vi "guangzi_16_up2.vi"() -> ()   [LabVIEW 2016]
uses:
  <vilib>/Utility/file.llb/Write To Spreadsheet File (DBL).vi
panel:
  in  "选项卡控件":T1(tab)
  in  "对数":bool
  out "MCS8Dat Error":i32
  out "通道数":i32
  out "Data 9":dbl[](graph)
  out "MCS8Dat Error 2":i32
  out "通道数 2":i32
  in  "对数 2":bool
  out "Data10":dbl[](graph)
  out "MCS8Dat Error 3":i32
  out "通道数 3":i32
  in  "对数 3":bool
  out "Data10 2":dbl[](graph)
  out "MCS8Dat Error 4":i32
  out "通道数 4":i32
  in  "对数 4":bool
  out "Data10 3":dbl[](graph)
  out "MCS8Dat Error 5":i32
  out "通道数 5":i32
  in  "对数 5":bool
  out "Data10 4":dbl[](graph)
  out "MCS8Dat Error 6":i32
  out "通道数 6":i32
  in  "对数 6":bool
  out "Data10 5":dbl[](graph)
  out "MCS8Dat Error 7":i32
  out "通道数 7":i32
  in  "对数 7":bool
  out "Data10 6":dbl[](graph)
  out "MCS8Dat Error 8":i32
  out "通道数 8":i32
  in  "对数 8":bool
  out "Data10 7":dbl[](graph)
  out "MCS8Dat Error 9":i32
  out "通道数 9":i32
  in  "对数 9":bool
  out "Data108":dbl[](graph)
  in  "对数 10":bool
  out "通道数 10":i32
  out "MCS8Dat Error 10":i32
  out "Data10 9":dbl[](graph)
  in  "对数 11":bool
  out "通道数 11":i32
  out "MCS8Dat Error 11":i32
  out "Data10 10":dbl[](graph)
  in  "对数 12":bool
  out "通道数 12":i32
  out "MCS8Dat Error 12":i32
  out "Data10 11":dbl[](graph)
  in  "对数 13":bool
  out "通道数 13":i32
  out "MCS8Dat Error 13":i32
  out "Data10 12":dbl[](graph)
  in  "对数 14":bool
  out "通道数 14":i32
  out "MCS8Dat Error 14":i32
  out "Data10 13":dbl[](graph)
  in  "对数 15":bool
  out "通道数 15":i32
  out "MCS8Dat Error 15":i32
  out "Data10 14":dbl[](graph)
  in  "对数 16":bool
  out "通道数 16":i32
  out "MCS8Dat Error 16":i32
  out "Data10 15":dbl[](graph)
  in  "切片值":i32
  out "切片图":u32[](graph)
  in  "采集开关":bool
  in  "子开关":bool
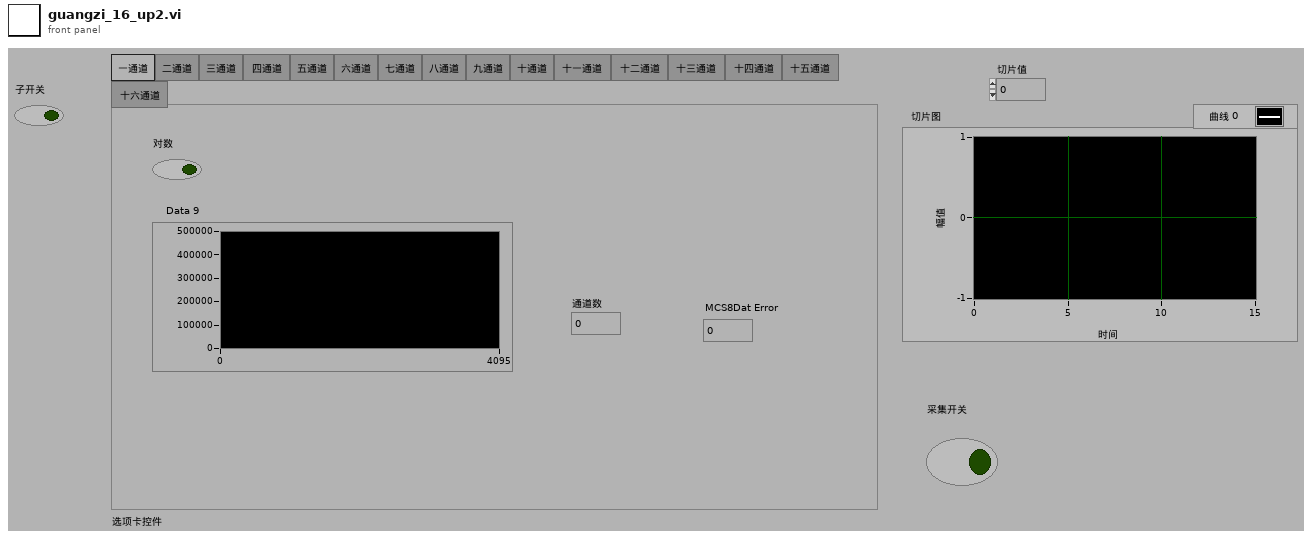
[diagram p1: front panel]
types:
  T1 = enum32{"一通道", "二通道", "三通道", "四通道 ", "五通道", "六通道", "七通道", "八通道", "九通道", "十通道", "十一通道 ", "十二通道 ", "十三通道 ", "十四通道 ", "十五通道 ", "十六通道 "}
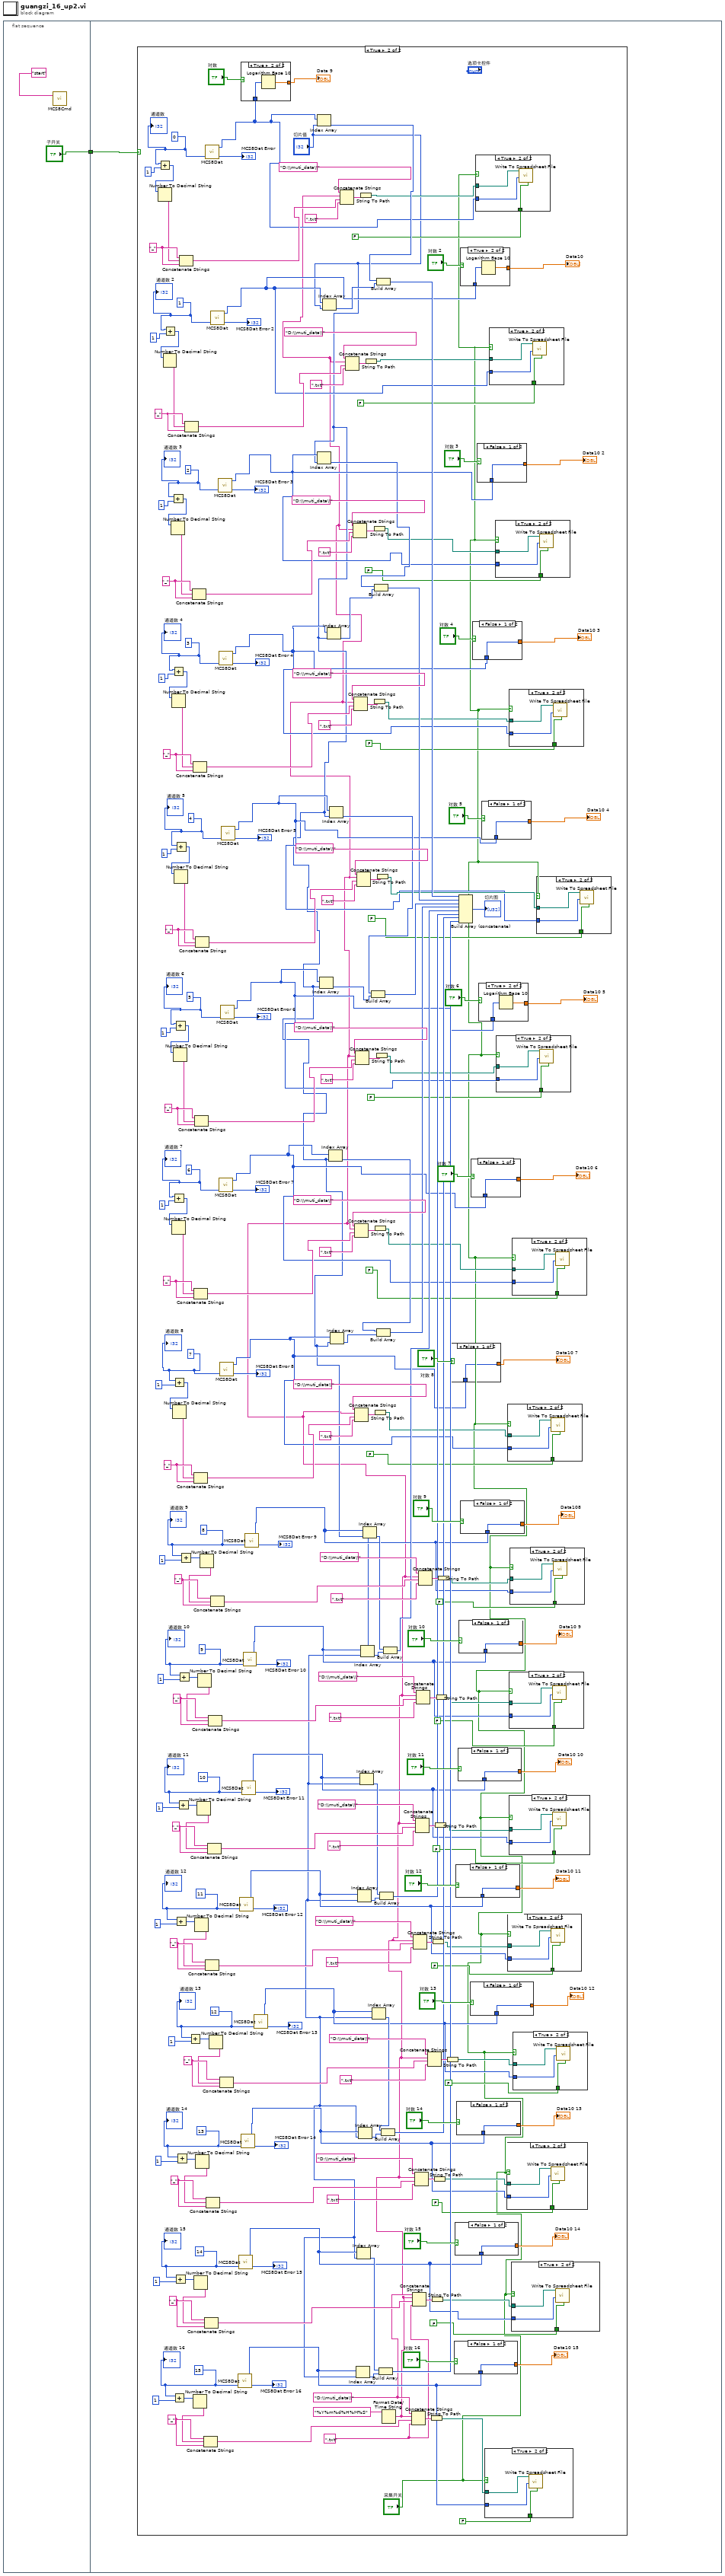
[diagram p0: block diagram]
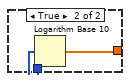
[diagram p19: hidden frame]
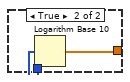
[diagram p20: hidden frame]
diagram:
  n1 = flat-sequence {
    tunnel: ["子开关"] -> w1
    tunnel: w1 -> [w4]
    frame #0 {
      n2 = call "MCS8Cmd.vi"("Command"="start") -> ()  [unwired: 2 in, 1 out]
    }
    frame #1 {
      n3 = case shown="True" w4 {
        frame False {
        }
        frame True {
          w6 = ".txt"
          w7 = "D:\\muti_data\\"
          w65 = "_"
          w69 = 15
          w75 = "_"
          w79 = 14
          w90 = "_"
          w94 = 13
          w102 = "_"
          w106 = 12
          w117 = "_"
          w121 = 11
          w129 = "_"
          w133 = 10
          w144 = "_"
          w148 = 9
          w156 = "_"
          w160 = 8
          w192 = 7
          w198 = "_"
          w202 = 6
          w208 = "_"
          w212 = 5
          w218 = "_"
          w222 = 4
          w228 = "_"
          w232 = 3
          w238 = "_"
          w242 = 2
          w248 = "_"
          w252 = 1
          w258 = "_"
          w262 = 0
          w268 = "_"
          n4 = Add(x=w262, y=1) -> (x+y=w264:i32)
          n5 = Number To Decimal String(number=w264) -> (decimal integer string=w267:string)  [unwired: 1 in]
          n6 = Add(x=w252, y=1) -> (x+y=w254:i32)
          n7 = Number To Decimal String(number=w254) -> (decimal integer string=w257:string)  [unwired: 1 in]
          n8 = Add(x=w242, y=1) -> (x+y=w244:i32)
          n9 = Number To Decimal String(number=w244) -> (decimal integer string=w247:string)  [unwired: 1 in]
          n10 = Add(x=w232, y=1) -> (x+y=w234:i32)
          n11 = Number To Decimal String(number=w234) -> (decimal integer string=w237:string)  [unwired: 1 in]
          n12 = Add(x=w202, y=1) -> (x+y=w204:i32)
          n13 = Number To Decimal String(number=w204) -> (decimal integer string=w207:string)  [unwired: 1 in]
          n14 = Add(x=w192, y=1) -> (x+y=w194:i32)
          n15 = Number To Decimal String(number=w194) -> (decimal integer string=w197:string)  [unwired: 1 in]
          n16 = Add(x=w69, y=1) -> (x+y=w70:i32)
          n17 = Add(x=w212, y=1) -> (x+y=w214:i32)
          n18 = Number To Decimal String(number=w214) -> (decimal integer string=w217:string)  [unwired: 1 in]
          n19 = Add(x=w79, y=1) -> (x+y=w80:i32)
          n20 = Add(x=w222, y=1) -> (x+y=w224:i32)
          n21 = Number To Decimal String(number=w224) -> (decimal integer string=w227:string)  [unwired: 1 in]
          n22 = Add(x=w121, y=1) -> (x+y=w122:i32)
          n23 = Add(x=w94, y=1) -> (x+y=w95:i32)
          n24 = Add(x=w133, y=1) -> (x+y=w134:i32)
          n25 = Add(x=w148, y=1) -> (x+y=w149:i32)
          n26 = Concatenate Strings(w268, w267, w268) -> (w266:string)
          n27 = Add(x=w160, y=1) -> (x+y=w161:i32)
          n28 = Concatenate Strings(w258, w257, w258) -> (w256:string)
          n29 = Add(x=w106, y=1) -> (x+y=w107:i32)
          n30 = Concatenate Strings(w248, w247, w248) -> (w246:string)
          n31 = Concatenate Strings(w238, w237, w238) -> (w236:string)
          n32 = Number To Decimal String(number=w70) -> (decimal integer string=w64:string)  [unwired: 1 in]
          n33 = Concatenate Strings(w208, w207, w208) -> (w206:string)
          n34 = Concatenate Strings(w198, w197, w198) -> (w196:string)
          n35 = Number To Decimal String(number=w80) -> (decimal integer string=w74:string)  [unwired: 1 in]
          n36 = Concatenate Strings(w218, w217, w218) -> (w216:string)
          n37 = Number To Decimal String(number=w122) -> (decimal integer string=w116:string)  [unwired: 1 in]
          n38 = Concatenate Strings(w228, w227, w228) -> (w226:string)
          n39 = Number To Decimal String(number=w95) -> (decimal integer string=w89:string)  [unwired: 1 in]
          n40 = Number To Decimal String(number=w134) -> (decimal integer string=w128:string)  [unwired: 1 in]
          n41 = Number To Decimal String(number=w149) -> (decimal integer string=w143:string)  [unwired: 1 in]
          n42 = Number To Decimal String(number=w161) -> (decimal integer string=w155:string)  [unwired: 1 in]
          n43 = Concatenate Strings(w65, w64, w65) -> (w62:string)
          n44 = Concatenate Strings(w75, w74, w75) -> (w73:string)
          n45 = call "MCS8Dat.vi"("Spectrum #"=w262) -> ("MCS8Dat Error"=→"MCS8Dat Error":i32, "Data"=w11:u32[])  [unwired: 2 in, 1 out]
          n46 = Concatenate Strings(w117, w116, w117) -> (w114:string)
          n47 = Concatenate Strings(w90, w89, w90) -> (w87:string)
          n48 = Concatenate Strings(w129, w128, w129) -> (w126:string)
          n49 = Concatenate Strings(w144, w143, w144) -> (w141:string)
          n50 = Number To Decimal String(number=w107) -> (decimal integer string=w101:string)  [unwired: 1 in]
          n51 = call "MCS8Dat.vi"("Spectrum #"=w252) -> ("MCS8Dat Error"=→"MCS8Dat Error 2":i32, "Data"=w14:u32[])  [unwired: 2 in, 1 out]
          n52 = Concatenate Strings(w156, w155, w156) -> (w153:string)
          n53 = call "MCS8Dat.vi"("Spectrum #"=w242) -> ("MCS8Dat Error"=→"MCS8Dat Error 3":i32, "Data"=w17:u32[])  [unwired: 2 in, 1 out]
          n54 = call "MCS8Dat.vi"("Spectrum #"=w232) -> ("MCS8Dat Error"=→"MCS8Dat Error 4":i32, "Data"=w20:u32[])  [unwired: 2 in, 1 out]
          n55 = call "MCS8Dat.vi"("Spectrum #"=w202) -> ("MCS8Dat Error"=→"MCS8Dat Error 7":i32, "Data"=w29:u32[])  [unwired: 2 in, 1 out]
          n56 = call "MCS8Dat.vi"("Spectrum #"=w192) -> ("MCS8Dat Error"=→"MCS8Dat Error 8":i32, "Data"=w32:u32[])  [unwired: 2 in, 1 out]
          n57 = Concatenate Strings(w102, w101, w102) -> (w99:string)
          n58 = call "MCS8Dat.vi"("Spectrum #"=w212) -> ("MCS8Dat Error"=→"MCS8Dat Error 6":i32, "Data"=w26:u32[])  [unwired: 2 in, 1 out]
          n59 = call "MCS8Dat.vi"("Spectrum #"=w222) -> ("MCS8Dat Error"=→"MCS8Dat Error 5":i32, "Data"=w23:u32[])  [unwired: 2 in, 1 out]
          n60 = call "MCS8Dat.vi"("Spectrum #"=w69) -> ("MCS8Dat Error"=→"MCS8Dat Error 16":i32, "Data"=w56:u32[])  [unwired: 2 in, 1 out]
          n61 = call "MCS8Dat.vi"("Spectrum #"=w79) -> ("MCS8Dat Error"=→"MCS8Dat Error 15":i32, "Data"=w53:u32[])  [unwired: 2 in, 1 out]
          n62 = call "MCS8Dat.vi"("Spectrum #"=w121) -> ("MCS8Dat Error"=→"MCS8Dat Error 12":i32, "Data"=w44:u32[])  [unwired: 2 in, 1 out]
          n63 = call "MCS8Dat.vi"("Spectrum #"=w94) -> ("MCS8Dat Error"=→"MCS8Dat Error 14":i32, "Data"=w50:u32[])  [unwired: 2 in, 1 out]
          n64 = case shown="True" "对数" {
            tunnel: w11 -> [w365 w366]
            tunnel: [w365 w367] -> w177
            frame False {
            }
            frame True {
              n65 = Logarithm Base 10(1:w366) -> (0:w367:dbl[])
            }
          }
          "Data 9" <- w177
          n66 = call "MCS8Dat.vi"("Spectrum #"=w133) -> ("MCS8Dat Error"=→"MCS8Dat Error 11":i32, "Data"=w41:u32[])  [unwired: 2 in, 1 out]
          n67 = call "MCS8Dat.vi"("Spectrum #"=w148) -> ("MCS8Dat Error"=→"MCS8Dat Error 10":i32, "Data"=w38:u32[])  [unwired: 2 in, 1 out]
          n68 = call "MCS8Dat.vi"("Spectrum #"=w160) -> ("MCS8Dat Error"=→"MCS8Dat Error 9":i32, "Data"=w35:u32[])  [unwired: 2 in, 1 out]
          n69 = call "MCS8Dat.vi"("Spectrum #"=w106) -> ("MCS8Dat Error"=→"MCS8Dat Error 13":i32, "Data"=w47:u32[])  [unwired: 2 in, 1 out]
          n70 = Index Array(array=w11, index="切片值") -> (element=w185:u32)
          n71 = Index Array(array=w17, index="切片值") -> (element=w187:u32)
          n72 = Index Array(array=w26, index="切片值") -> (element=w189:u32)
          n73 = Index Array(array=w14, index="切片值") -> (element=w184:u32)
          n74 = Index Array(array=w20, index="切片值") -> (element=w186:u32)
          n75 = Index Array(array=w29, index="切片值") -> (element=w190:u32)
          n76 = Index Array(array=w23, index="切片值") -> (element=w188:u32)
          n77 = Index Array(array=w32, index="切片值") -> (element=w191:u32)
          n78 = Index Array(array=w56, index="切片值") -> (element=w60:u32)
          n79 = Index Array(array=w53, index="切片值") -> (element=w59:u32)
          n80 = Index Array(array=w44, index="切片值") -> (element=w110:u32)
          n81 = Index Array(array=w50, index="切片值") -> (element=w83:u32)
          n82 = Index Array(array=w41, index="切片值") -> (element=w111:u32)
          n83 = Index Array(array=w38, index="切片值") -> (element=w137:u32)
          n84 = Index Array(array=w35, index="切片值") -> (element=w138:u32)
          n85 = Build Array(w188, w189) -> (w181:u32[])
          n86 = Index Array(array=w47, index="切片值") -> (element=w84:u32)
          n87 = Build Array(w187, w186) -> (w182:u32[])
          n88 = Build Array(w190, w191) -> (w180:u32[])
          n89 = Build Array(w185, w184) -> (w183:u32[])
          n90 = Build Array(w59, w60) -> (w58:u32[])
          n91 = Build Array(w111, w110) -> (w109:u32[])
          n92 = Build Array(w84, w83) -> (w82:u32[])
          n93 = Format Date/Time String(time format string (%c)="%Y%m%d%H%M%S") -> (date/time string=w5:string)  [unwired: 2 in]
          n94 = Concatenate Strings("D:\\muti_data\\", w5, w266, ".txt") -> (w270:string)
          n95 = Concatenate Strings("D:\\muti_data\\", w5, w256, ".txt") -> (w260:string)
          n96 = Concatenate Strings("D:\\muti_data\\", w5, w246, ".txt") -> (w250:string)
          n97 = Concatenate Strings("D:\\muti_data\\", w5, w236, ".txt") -> (w240:string)
          n98 = Concatenate Strings("D:\\muti_data\\", w5, w206, ".txt") -> (w210:string)
          n99 = Concatenate Strings("D:\\muti_data\\", w5, w196, ".txt") -> (w200:string)
          n100 = Concatenate Strings("D:\\muti_data\\", w5, w216, ".txt") -> (w220:string)
          n101 = Concatenate Strings("D:\\muti_data\\", w5, w226, ".txt") -> (w230:string)
          n102 = String To Path(string=w270) -> (path=w12:path)
          n103 = String To Path(string=w260) -> (path=w15:path)
          n104 = String To Path(string=w250) -> (path=w18:path)
          n105 = String To Path(string=w240) -> (path=w21:path)
          n106 = String To Path(string=w210) -> (path=w30:path)
          n107 = String To Path(string=w200) -> (path=w33:path)
          n108 = String To Path(string=w220) -> (path=w27:path)
          n109 = String To Path(string=w230) -> (path=w24:path)
          n110 = Build Array(w138, w137) -> (w136:u32[])
          n111 = Concatenate Strings(w7, w5, w62, w6) -> (w61:string)
          n112 = Concatenate Strings(w7, w5, w73, w6) -> (w72:string)
          n113 = Concatenate Strings("D:\\muti_data\\", w5, w114, ".txt") -> (w112:string)
          n114 = Concatenate Strings("D:\\muti_data\\", w5, w87, ".txt") -> (w85:string)
          n115 = Concatenate Strings("D:\\muti_data\\", w5, w126, ".txt") -> (w124:string)
          n116 = Concatenate Strings("D:\\muti_data\\", w5, w141, ".txt") -> (w139:string)
          n117 = Concatenate Strings("D:\\muti_data\\", w5, w153, ".txt") -> (w151:string)
          n118 = Concatenate Strings("D:\\muti_data\\", w5, w99, ".txt") -> (w97:string)
          n119 = String To Path(string=w61) -> (path=w57:path)
          n120 = String To Path(string=w72) -> (path=w54:path)
          n121 = String To Path(string=w112) -> (path=w45:path)
          n122 = String To Path(string=w85) -> (path=w49:path)
          n123 = String To Path(string=w124) -> (path=w42:path)
          n124 = String To Path(string=w139) -> (path=w39:path)
          n125 = String To Path(string=w151) -> (path=w36:path)
          n126 = String To Path(string=w97) -> (path=w48:path)
          n127 = case shown="False" "对数 8" {
            tunnel: w32 -> [w344 w346]
            tunnel: [w344 w345] -> w163
            frame False {
            }
            frame True {
              n128 = Logarithm Base 10(1:w346) -> (0:w345:dbl[])
            }
          }
          "Data10 7" <- w163
          n129 = case shown="False" "对数 16" {
            tunnel: w56 -> [w320 w322]
            tunnel: [w320 w321] -> w66
            frame False {
            }
            frame True {
              n130 = Logarithm Base 10(1:w322) -> (0:w321:dbl[])
            }
          }
          "Data10 15" <- w66
          n131 = case shown="False" "对数 15" {
            tunnel: w53 -> [w323 w325]
            tunnel: [w323 w324] -> w76
            frame False {
            }
            frame True {
              n132 = Logarithm Base 10(1:w325) -> (0:w324:dbl[])
            }
          }
          "Data10 14" <- w76
          n133 = case shown="False" "对数 12" {
            tunnel: w44 -> [w332 w334]
            tunnel: [w332 w333] -> w118
            frame False {
            }
            frame True {
              n134 = Logarithm Base 10(1:w334) -> (0:w333:dbl[])
            }
          }
          "Data10 11" <- w118
          n135 = case shown="False" "对数 14" {
            tunnel: w50 -> [w326 w328]
            tunnel: [w326 w327] -> w91
            frame False {
            }
            frame True {
              n136 = Logarithm Base 10(1:w328) -> (0:w327:dbl[])
            }
          }
          "Data10 13" <- w91
          n137 = case shown="False" "对数 11" {
            tunnel: w41 -> [w335 w337]
            tunnel: [w335 w336] -> w130
            frame False {
            }
            frame True {
              n138 = Logarithm Base 10(1:w337) -> (0:w336:dbl[])
            }
          }
          "Data10 10" <- w130
          n139 = Build Array (concatenate)(w183, w182, w181, w180, w136, w109, w82, w58) -> (→"切片图":u32[])
          n140 = case shown="False" "对数 10" {
            tunnel: w38 -> [w338 w340]
            tunnel: [w338 w339] -> w145
            frame False {
            }
            frame True {
              n141 = Logarithm Base 10(1:w340) -> (0:w339:dbl[])
            }
          }
          "Data10 9" <- w145
          n142 = case shown="True" "对数 2" {
            tunnel: w14 -> [w362 w364]
            tunnel: [w362 w363] -> w175
            frame False {
            }
            frame True {
              n143 = Logarithm Base 10(1:w364) -> (0:w363:dbl[])
            }
          }
          "Data10" <- w175
          n144 = case shown="False" "对数 9" {
            tunnel: w35 -> [w341 w343]
            tunnel: [w341 w342] -> w157
            frame False {
            }
            frame True {
              n145 = Logarithm Base 10(1:w343) -> (0:w342:dbl[])
            }
          }
          "Data108" <- w157
          n146 = case shown="False" "对数 13" {
            tunnel: w47 -> [w329 w331]
            tunnel: [w329 w330] -> w103
            frame False {
            }
            frame True {
              n147 = Logarithm Base 10(1:w331) -> (0:w330:dbl[])
            }
          }
          "Data10 12" <- w103
          n148 = case shown="False" "对数 7" {
            tunnel: w29 -> [w347 w349]
            tunnel: [w347 w348] -> w165
            frame False {
            }
            frame True {
              n149 = Logarithm Base 10(1:w349) -> (0:w348:dbl[])
            }
          }
          "Data10 6" <- w165
          n150 = case shown="False" "对数 4" {
            tunnel: w20 -> [w356 w358]
            tunnel: [w356 w357] -> w171
            frame False {
            }
            frame True {
              n151 = Logarithm Base 10(1:w358) -> (0:w357:dbl[])
            }
          }
          "Data10 3" <- w171
          n152 = case shown="True" "采集开关" {
            tunnel: w12 -> [_ w274]
            tunnel: w11 -> [_ w273]
            tunnel: FALSE -> [_ w272]
            frame False {
            }
            frame True {
              n153 = call-poly <vilib>:"Write To Spreadsheet File.vi"("transpose? (no:F)"=w272, "1D data"=w273, "file path (dialog if empty)"=w274) -> ()  [unwired: 5 in, 1 out]
            }
          }
          n154 = case shown="False" "对数 3" {
            tunnel: w17 -> [w359 w361]
            tunnel: [w359 w360] -> w173
            frame False {
            }
            frame True {
              n155 = Logarithm Base 10(1:w361) -> (0:w360:dbl[])
            }
          }
          "Data10 2" <- w173
          n156 = case shown="True" "对数 6" {
            tunnel: w26 -> [w350 w352]
            tunnel: [w350 w351] -> w167
            frame False {
            }
            frame True {
              n157 = Logarithm Base 10(1:w352) -> (0:w351:dbl[])
            }
          }
          "Data10 5" <- w167
          n158 = case shown="False" "对数 5" {
            tunnel: w23 -> [w353 w355]
            tunnel: [w353 w354] -> w169
            frame False {
            }
            frame True {
              n159 = Logarithm Base 10(1:w355) -> (0:w354:dbl[])
            }
          }
          "Data10 4" <- w169
          n160 = case shown="True" "采集开关" {
            tunnel: w57 -> [_ w319]
            tunnel: w56 -> [_ w318]
            tunnel: FALSE -> [_ w317]
            frame False {
            }
            frame True {
              n161 = call-poly <vilib>:"Write To Spreadsheet File.vi"("transpose? (no:F)"=w317, "1D data"=w318, "file path (dialog if empty)"=w319) -> ()  [unwired: 5 in, 1 out]
            }
          }
          n162 = case shown="True" "采集开关" {
            tunnel: w15 -> [_ w277]
            tunnel: w14 -> [_ w276]
            tunnel: FALSE -> [_ w275]
            frame False {
            }
            frame True {
              n163 = call-poly <vilib>:"Write To Spreadsheet File.vi"("transpose? (no:F)"=w275, "1D data"=w276, "file path (dialog if empty)"=w277) -> ()  [unwired: 5 in, 1 out]
            }
          }
          n164 = case shown="True" "采集开关" {
            tunnel: w18 -> [_ w280]
            tunnel: w17 -> [_ w279]
            tunnel: FALSE -> [_ w278]
            frame False {
            }
            frame True {
              n165 = call-poly <vilib>:"Write To Spreadsheet File.vi"("transpose? (no:F)"=w278, "1D data"=w279, "file path (dialog if empty)"=w280) -> ()  [unwired: 5 in, 1 out]
            }
          }
          n166 = case shown="True" "采集开关" {
            tunnel: w27 -> [_ w289]
            tunnel: w26 -> [_ w288]
            tunnel: FALSE -> [_ w287]
            frame False {
            }
            frame True {
              n167 = call-poly <vilib>:"Write To Spreadsheet File.vi"("transpose? (no:F)"=w287, "1D data"=w288, "file path (dialog if empty)"=w289) -> ()  [unwired: 5 in, 1 out]
            }
          }
          n168 = case shown="True" "采集开关" {
            tunnel: w49 -> [_ w313]
            tunnel: w50 -> [_ w312]
            tunnel: FALSE -> [_ w311]
            frame False {
            }
            frame True {
              n169 = call-poly <vilib>:"Write To Spreadsheet File.vi"("transpose? (no:F)"=w311, "1D data"=w312, "file path (dialog if empty)"=w313) -> ()  [unwired: 5 in, 1 out]
            }
          }
          n170 = case shown="True" "采集开关" {
            tunnel: w33 -> [_ w295]
            tunnel: w32 -> [_ w294]
            tunnel: FALSE -> [_ w293]
            frame False {
            }
            frame True {
              n171 = call-poly <vilib>:"Write To Spreadsheet File.vi"("transpose? (no:F)"=w293, "1D data"=w294, "file path (dialog if empty)"=w295) -> ()  [unwired: 5 in, 1 out]
            }
          }
          n172 = case shown="True" "采集开关" {
            tunnel: w45 -> [_ w307]
            tunnel: w44 -> [_ w306]
            tunnel: FALSE -> [_ w305]
            frame False {
            }
            frame True {
              n173 = call-poly <vilib>:"Write To Spreadsheet File.vi"("transpose? (no:F)"=w305, "1D data"=w306, "file path (dialog if empty)"=w307) -> ()  [unwired: 5 in, 1 out]
            }
          }
          n174 = case shown="True" "采集开关" {
            tunnel: w39 -> [_ w301]
            tunnel: w38 -> [_ w300]
            tunnel: FALSE -> [_ w299]
            frame False {
            }
            frame True {
              n175 = call-poly <vilib>:"Write To Spreadsheet File.vi"("transpose? (no:F)"=w299, "1D data"=w300, "file path (dialog if empty)"=w301) -> ()  [unwired: 5 in, 1 out]
            }
          }
          n176 = case shown="True" "采集开关" {
            tunnel: w42 -> [_ w304]
            tunnel: w41 -> [_ w303]
            tunnel: FALSE -> [_ w302]
            frame False {
            }
            frame True {
              n177 = call-poly <vilib>:"Write To Spreadsheet File.vi"("transpose? (no:F)"=w302, "1D data"=w303, "file path (dialog if empty)"=w304) -> ()  [unwired: 5 in, 1 out]
            }
          }
          n178 = case shown="True" "采集开关" {
            tunnel: w21 -> [_ w283]
            tunnel: w20 -> [_ w282]
            tunnel: FALSE -> [_ w281]
            frame False {
            }
            frame True {
              n179 = call-poly <vilib>:"Write To Spreadsheet File.vi"("transpose? (no:F)"=w281, "1D data"=w282, "file path (dialog if empty)"=w283) -> ()  [unwired: 5 in, 1 out]
            }
          }
          n180 = case shown="True" "采集开关" {
            tunnel: w36 -> [_ w298]
            tunnel: w35 -> [_ w297]
            tunnel: FALSE -> [_ w296]
            frame False {
            }
            frame True {
              n181 = call-poly <vilib>:"Write To Spreadsheet File.vi"("transpose? (no:F)"=w296, "1D data"=w297, "file path (dialog if empty)"=w298) -> ()  [unwired: 5 in, 1 out]
            }
          }
          n182 = case shown="True" "采集开关" {
            tunnel: w54 -> [_ w316]
            tunnel: w53 -> [_ w315]
            tunnel: FALSE -> [_ w314]
            frame False {
            }
            frame True {
              n183 = call-poly <vilib>:"Write To Spreadsheet File.vi"("transpose? (no:F)"=w314, "1D data"=w315, "file path (dialog if empty)"=w316) -> ()  [unwired: 5 in, 1 out]
            }
          }
          n184 = case shown="True" "采集开关" {
            tunnel: w30 -> [_ w292]
            tunnel: w29 -> [_ w291]
            tunnel: FALSE -> [_ w290]
            frame False {
            }
            frame True {
              n185 = call-poly <vilib>:"Write To Spreadsheet File.vi"("transpose? (no:F)"=w290, "1D data"=w291, "file path (dialog if empty)"=w292) -> ()  [unwired: 5 in, 1 out]
            }
          }
          n186 = case shown="True" "采集开关" {
            tunnel: w48 -> [_ w310]
            tunnel: w47 -> [_ w309]
            tunnel: FALSE -> [_ w308]
            frame False {
            }
            frame True {
              n187 = call-poly <vilib>:"Write To Spreadsheet File.vi"("transpose? (no:F)"=w308, "1D data"=w309, "file path (dialog if empty)"=w310) -> ()  [unwired: 5 in, 1 out]
            }
          }
          n188 = case shown="True" "采集开关" {
            tunnel: w24 -> [_ w286]
            tunnel: w23 -> [_ w285]
            tunnel: FALSE -> [_ w284]
            frame False {
            }
            frame True {
              n189 = call-poly <vilib>:"Write To Spreadsheet File.vi"("transpose? (no:F)"=w284, "1D data"=w285, "file path (dialog if empty)"=w286) -> ()  [unwired: 5 in, 1 out]
            }
          }
          "通道数" <- w262
          "通道数 2" <- w252
          "通道数 3" <- w242
          "通道数 4" <- w232
          "通道数 5" <- w222
          "通道数 6" <- w212
          "通道数 7" <- w202
          "通道数 8" <- w192
          "通道数 9" <- w160
          "通道数 10" <- w148
          "通道数 11" <- w133
          "通道数 12" <- w121
          "通道数 13" <- w106
          "通道数 14" <- w94
          "通道数 15" <- w79
          "通道数 16" <- w69
        }
      }
    }
  }
